vi "VISA IDN SX199 Fix.vi"(6 "Manufacturer in":string, 7 "Revision in":string, 8 "error in (no error)":errorcluster {"code" format="%.0x"}, 9 "Info in":string, 10 "Model in":string, 11 "VISA Resource Name":refnum<visa-resource-name>) -> (0 "error out":errorcluster {"code" format="%.0x"}, 1 "Extra Info":i32[](array[numeric]), 2 "Devices":T1[](array[typedef]) {"Status" format="%.0x"}, 3 "dup VISA Session":refnum<visa-resource-name>)   [LabVIEW 2020]
uses:
  New NML Data Acq/Sub Controls/Instrument IDN.ctl
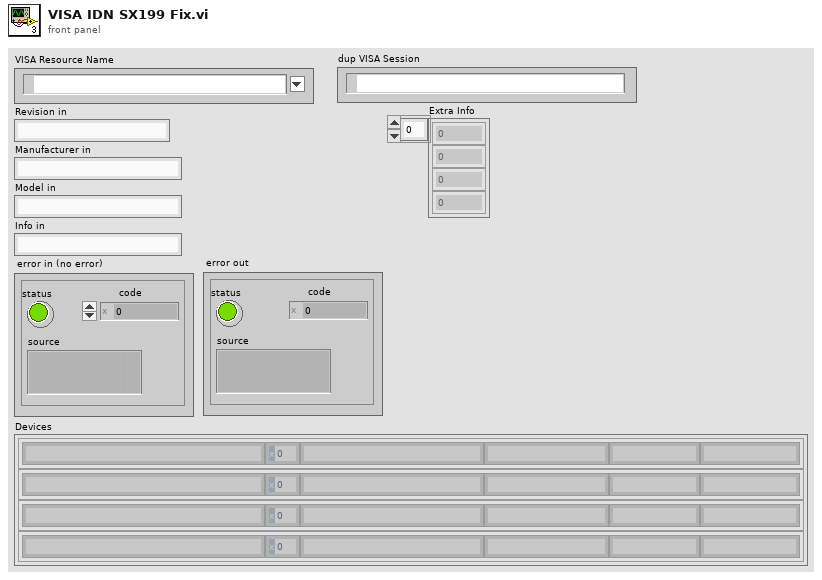
[diagram p1: front panel]
types:
  T1 = typedef "Instrument IDN.ctl" = cluster{"VISA Address":string, "Status":u16, "Manufacturer":string, "Model":string, "Info":string, "Info 2":string, "Misc Data":variant}
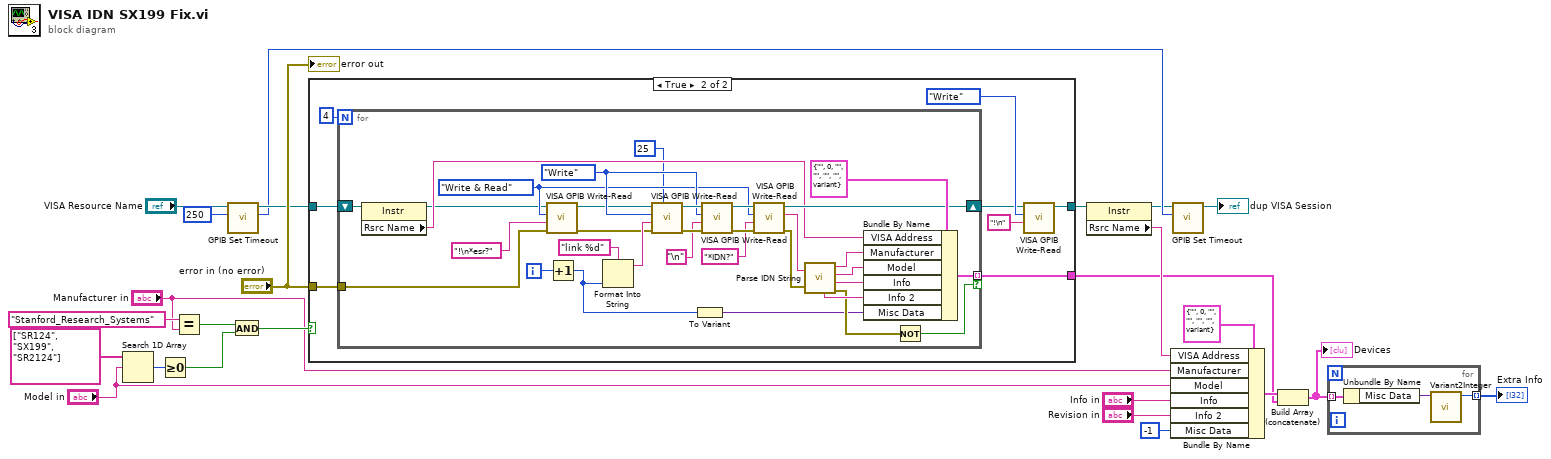
[diagram p0: block diagram]
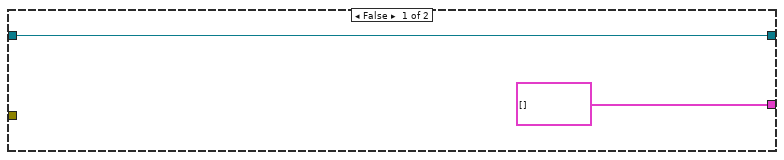
[diagram p2: hidden frame]
diagram:
  n1 = Search 1D Array(1D array=string[] ["SR124", "SX199", "SR2124"], element="Model in") -> (index of element=w5:i32)  [unwired: 1 in]
  n2 = Greater Or Equal To 0?(x=w5) -> (x >= 0?=w4:bool)
  n3 = Equal?(x="Stanford_Research_Systems" ("y"), y="Manufacturer in") -> (x = y?=w23:bool)
  n4 = call "GPIB Set Timeout.vi"("Timeout"=u32 250, "VISA resource name"="VISA Resource Name") -> ("Old Timeout"=w14:u32, "dup VISA resource name"=w18:refnum<visa-resource-name>)  [unwired: 3 in, 1 out]
  n5 = And(x=w23, y=w4) -> (x .and. y?=w25:bool)
  n6 = case shown="True" w25 {
    tunnel: "error in (no error)" -> [_ w33]
    tunnel: [T1[] [] w32] -> w10
    tunnel: w18 -> [w26 w34]
    tunnel: [w26 w29] -> w2
    frame False {
    }
    frame True {
      n7 = for {
        N: 4 -> [_]
        tunnel: [w51] -> w32 mode=indexing if=w47
        shift-right: [w50] -> w28
        shift-left: w34 -> [w37]
        tunnel: w33 -> [w43]
        i -> [w67]
        w45 = enum16{"Write", "Read", "Write & Read"}."Write & Read" ("Action")
        w46 = enum16{"Write", "Read", "Write & Read"}."Write" ("Action")
        n8 = property class="Instr"(reference=w37) -> (reference out=w36:refnum<visa-resource-name>, "Rsrc Name"=w49:string)  [unwired: 1 in, 1 out]
        n9 = call "VISA GPIB Write-Read.vi"("error in (no error)"=w43, "Command"="!\n*esr?" ("format string"), "Action"=w45, "VISA resource name"=w36) -> ("error out"=w42:errorcluster, "dup VISA Session"=w44:refnum<visa-resource-name>)  [unwired: 4 in, 2 out]
        n10 = Increment(x=w67) -> (x+1=w40:i32)
        n11 = Format Into String(format string="link %d", w40) -> (resulting string=w65:string)  [unwired: 2 in, 1 out]
        n12 = call "VISA GPIB Write-Read.vi"("Wait (ms)"=u32 25, "error in (no error)"=w42, "Command"=w65, "Action"=w46, "VISA resource name"=w44) -> ("error out"=w63:errorcluster, "dup VISA Session"=w62:refnum<visa-resource-name>)  [unwired: 3 in, 2 out]
        n13 = To Variant(anything=w40) -> (Variant=w38:variant)
        n14 = call "VISA GPIB Write-Read.vi"("error in (no error)"=w63, "Command"="\n", "Action"=w46, "VISA resource name"=w62) -> ("error out"=w60:errorcluster, "dup VISA Session"=w59:refnum<visa-resource-name>)  [unwired: 4 in, 2 out]
        n15 = call "VISA GPIB Write-Read.vi"("error in (no error)"=w60, "Command"="*IDN?" ("write buffer (\"\")"), "Action"=w45, "VISA resource name"=w59) -> ("error out"=w57:errorcluster, "String Returned"=w56:string, "dup VISA Session"=w50:refnum<visa-resource-name>)  [unwired: 4 in, 1 out]
        n16 = call "Parse IDN String.vi"("error in (no error)"=w57, "IDN String"=w56) -> ("error out"=w48:errorcluster, "Info"=w55:string, "Model"=w54:string, "Manufacturer"=w52:string, "Revision"=w53:string)
        n17 = Bundle By Name(cluster=T1 {"VISA Address"="", "Status"=0, "Manufacturer"="", "Model"="", "Info"="", "Info 2"="", "Misc Data"=variant} ("Instrument List"), "VISA Address"=w49, "Manufacturer"=w52, "Model"=w54, "Info"=w55, "Info 2"=w53, "Misc Data"=w38) -> (w51:T1)
        n18 = Not(x=w48) -> (.not. x?=w47:bool)
      }
      n19 = call "VISA GPIB Write-Read.vi"("Command"="!\n", "Action"=enum16{"Write", "Read", "Write & Read"}."Write", "VISA resource name"=w28) -> ("dup VISA Session"=w29:refnum<visa-resource-name>)  [unwired: 5 in, 3 out]
    }
  }
  n20 = property class="Instr"(reference=w2) -> (reference out=w1:refnum<visa-resource-name>, "Rsrc Name"=w11:string)  [unwired: 1 in, 1 out]
  n21 = Bundle By Name(cluster=T1 {"VISA Address"="", "Status"=0, "Manufacturer"="", "Model"="", "Info"="", "Info 2"="", "Misc Data"=variant} ("Instrument List"), "VISA Address"=w11, "Manufacturer"="Manufacturer in", "Model"="Model in", "Info"="Info in", "Info 2"="Revision in", "Misc Data"=-1) -> (w12:T1)
  n22 = call "GPIB Set Timeout.vi"("Timeout"=w14, "VISA resource name"=w1) -> ("dup VISA resource name"=→"dup VISA Session":refnum<visa-resource-name>)  [unwired: 3 in, 2 out]
  n23 = Build Array (concatenate)(w12, w10) -> (w8:T1[])
  "Devices" <- w8
  n24 = for {
    tunnel: w8 -> [w70] mode=indexing
    tunnel: [w69] -> w7 mode=indexing
    n25 = Unbundle By Name(w70) -> ("Misc Data"=w68:variant)
    n26 = call "Variant2Integer.vi"("Variant"=w68) -> ("data"=w69:i32)  [unwired: 9 in, 1 out]
  }
  "Extra Info" <- w7
  "error out" <- "error in (no error)"
